vi "Method_Const.vi"(4 "Value":ext, 5 "Value A":refnum<class "Abs_Extended Float.lvclass">) -> (1 "Result":refnum<class "Abs_Boolean.lvclass">)   [LabVIEW 2021, in "Not Equal_EXT.lvclass"]
uses:
  Not Equal_EXT.lvclass
  Abs_Types/Extended Float/Abs_Extended Float.lvclass
  C:/Program Files (x86)/National Instruments/LabVIEW 2021/vi.lib/TSA/Abstract Data Classes/Abs_Types/Numeric/Abs_Numeric.lvclass
  Abs_Types/Boolean/Abs_Boolean.lvclass
  C:/TSA/LV_Abstract/Source/Functions/Support/Compare/Two Term/EXT/AbsComp_Two Term_EXT.lvclass
  C:/Program Files (x86)/National Instruments/LabVIEW 2021/vi.lib/TSA/Abstract Data Classes/Abs_Types/Boolean/Abs_Boolean.lvclass
  Support/Compare/Two Term/EXT/AbsComp_Two Term_EXT.lvclass/AbsComp_Two Term_EXT.ctl
  Support/Compare/Two Term/EXT/Properties/Write Numeric A.vi
  Support/Compare/Two Term/EXT/Properties/Write Numeric B.vi
  Constants/Support/EXT/Const_EXT.lvclass
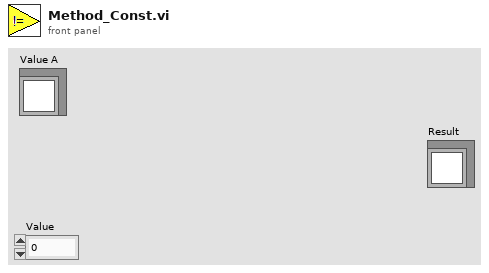
[diagram p1: front panel]
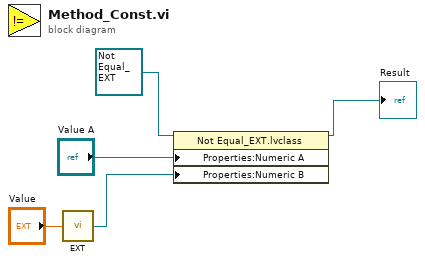
[diagram p0: block diagram]
diagram:
  n1 = call "EXT.vi"("Value"="Value") -> ("Constant"=w2:refnum<class "Abs_Extended Float.lvclass">)  [unwired: 4 in]
  n2 = property class="Not Equal_EXT.lvclass"(reference=refnum<class "Not Equal_EXT.lvclass"> refnum ("Greater 0_U64.lvclass"), "Properties:Numeric A"="Value A", "Properties:Numeric B"=w2) -> (reference out=→"Result":refnum<class "Not Equal_EXT.lvclass">)  [unwired: 1 in, 1 out]
